vi "Get Module Direction.vi"(8 "error in (no error)":errorcluster, 11 "Module in":refnum<class "Module.lvclass">) -> (0 "error out":errorcluster, 2 "Direction":enum16{"Input", "Output"}(ring), 3 "Module out":refnum<class "Module.lvclass">)   [LabVIEW 2015, in "Module.lvclass"]
uses:
  Module.lvclass
  Module Configuration.ctl
  Module.lvclass/Module.ctl
  VI/Module Loop/Module Loop.lvclass
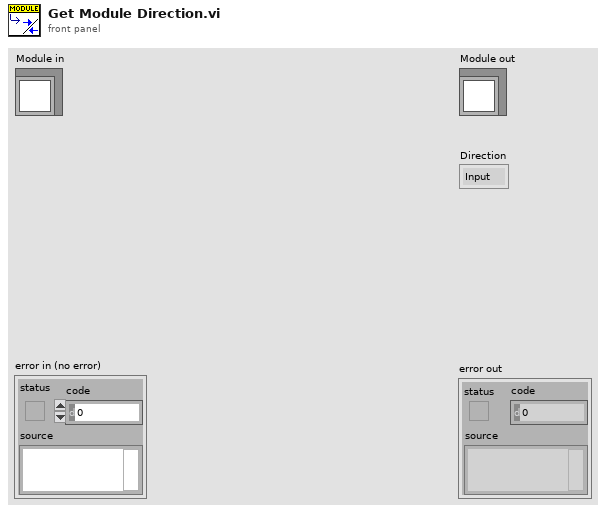
[diagram p1: front panel]
types:
  T1 = typedef "Module Loop.lvclass/Module Configuration.ctl" = cluster{"Type":string, "Direction":string, "Speed":string, "Channels":string, "FXP Type":string}
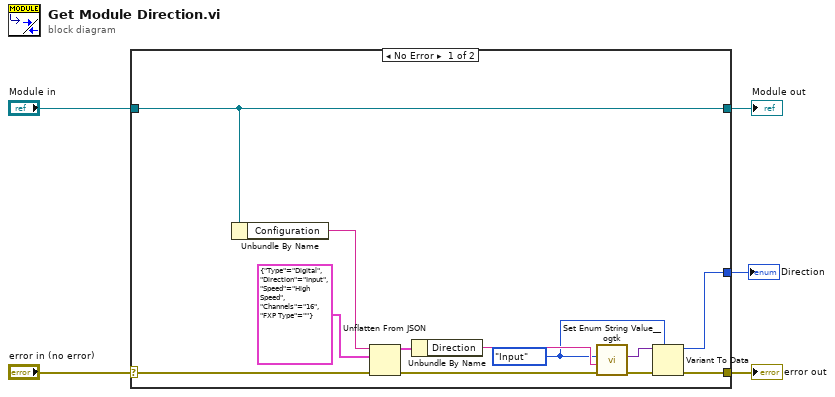
[diagram p0: block diagram]
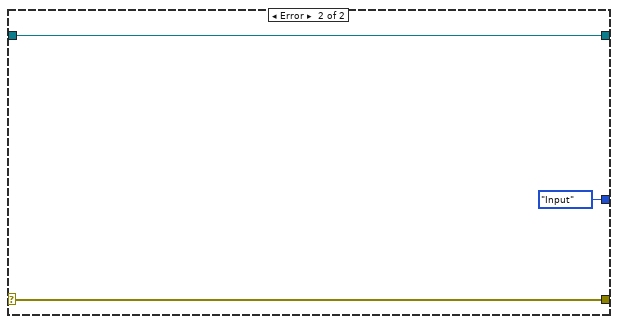
[diagram p2: hidden frame]
diagram:
  n1 = case shown="No Error" "error in (no error)" {
    selector: "error in (no error)" -> [w15 w20]
    tunnel: [w9 w20] -> w4
    tunnel: [w17 w19] -> w2
    tunnel: "Module in" -> [w17 w19]
    tunnel: [w7 enum16{"Input", "Output"}."Input" ("Direction")] -> w1
    frame No Error {
      w6 = enum16{"Input", "Output"}."Input" ("Direction")
      n2 = Unbundle By Name(w17) -> ("Configuration"=w16:string)
      n3 = Unflatten From JSON(JSON string=w16, type and defaults=T1 {"Type"="Digital", "Direction"="Input", "Speed"="High Speed", "Channels"="16", "FXP Type"=""} ("Cluster"), error in (no error)=w15) -> (value=w13:T1, error out=w10:errorcluster)  [unwired: 4 in]
      n4 = Unbundle By Name(w13) -> ("Direction"=w8:string)
      n5 = call <userlib>:"Set Enum String Value__ogtk.vi"("error in (no error)"=w10, "String Value"=w8, "Default Enum Value"=w6) -> ("error out"=w12:errorcluster, "Enum"=w11:variant)  [unwired: 7 in]
      n6 = Variant To Data(error in=w12, type=w6, Variant=w11) -> (data=w7:enum16{"Input", "Output"}, error out=w9:errorcluster)
    }
    frame Error {
    }
  }
  "error out" <- w4
  "Module out" <- w2
  "Direction" <- w1
